vi "Names.vi"() -> ()   [LabVIEW 2017, in "NI 272x Resistive Simulation Custom Device Shared.lvlib"]
uses:
  NI 272x Resistive Simulation Custom Device Shared.lvlib
panel:
  in  "group.diagnostics":string="group.diagnostics"
  in  "group.banks":string="group.banks"
  in  "group.desired":string="group.desired"
  in  "group.actual":string="group.actual"
  in  "Main page GUID":string="21b70d88-f326-4fa7-aab6-5b7b3a71cf29"
  in  "CompiledEngineData":string="CompiledEngineData"
  in  "Bank Connection Channel GUID":string="8C90FD46-3984-847B-99F6-649F225F3DB0"
  in  "Status Channel GUID":string="66F3C718-DF01-8B47-2232-60AEE9B9D6E4"
  in  "UpdateRate":string="UpdateRate"
  in  "RTDR0":string="RTDR0"
  in  "RTDC":string="RTDC"
  in  "RTDB":string="RTDB"
  in  "RTDA":string="RTDA"
  in  "Status Section GUID":string="E2E4C904-8981-DDC5-8A2C-603AEAD521EE"
  in  "Desired Value GUID":string="37e188a1-b520-407b-93e2-e3106e977a09"
  in  "Actual Value GUID":string="04a7b86c2-779e-4db5-ad36-60fe8eaba580"
  in  "Section GUID":string="76c539f1-1459-41eb-b62b-d9b6dff6cc8a"
  in  "Chan Type":string="Resource Name"
  in  "Channel  #":string="Channel Num"
  in  "Temperature constants":string="Temperature Constants"
  in  "Channel Mode":string="Channel Mode"
  in  "# Chan Tot":string="Num Chan"
  in  "Resource Name":string="Resource Name"
  # "resource name is \nthe name of the \ndevice in MAX"
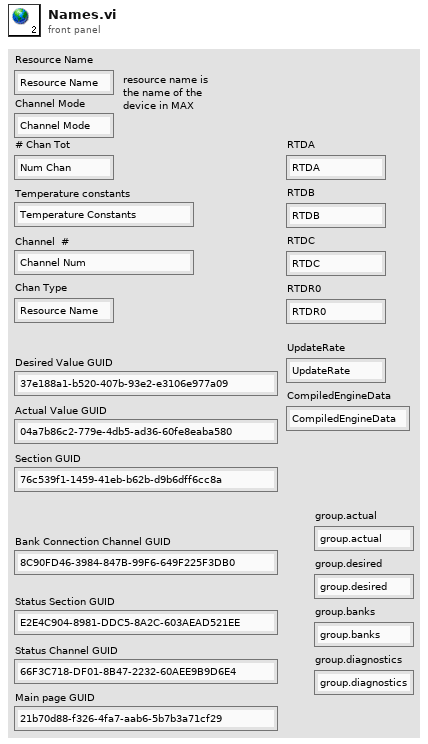
[diagram p1: front panel]
diagram:
